vi "AR Drone - Simple Video + Simple nav.vi"() -> ()   [LabVIEW 2014]
doc: "Very simple example showing how to use the base VIs to control the AR Drone and receive and display video data."
uses:
  Others (.ctl)/Control cluster.ctl
  <vilib>/LVH/AR Drone Toolkit/Decode NavData/Typedefs/NavData Demo.ctl
  Global.vi
  <vilib>/LVH/AR Drone Toolkit/AR Drone.lvlib
panel:
  in  "video refresh (ms)":u32
  out "Refesh Rate Video Loop (ms) 2":u32
  in  "Video":bool
  out "Refesh Rate (ms)":u32
  out "Hover":bool
  in  "Tab Control":enum32{"Page 1", "Page 2"}(tab)=enum."Page 2"
  out "Image":T1(plugin-control)
  out "Video Stream 2":picture
  in  "Manual":bool=TRUE
  in  "Takeoff/Land":bool
  in  "Setup Parameters":T2={"Drone IP address"="192.168.1.1", "Home IP address"="192.168.1.2", "Flight Mode"=enum."INDOOR MODE", "Mounted Hull"=enum."INDOOR HULL", "Video Camera"=0, "Max Altitude (m)"=3.0, "Max Pitch and Roll Angle (deg)"=10.0, "Max Vertical Speed (m/s)"=0.7, "Max Yaw Speed (deg/s)"=100.0} {"Video Camera" items=["Bottom Camera"=1, "Front Camera"=0, "Front in Bottom"=3, "Bottom in Front"=2]}
  in  "stop":bool
  in  "milliseconds to wait":u32=5
  out "ctr+nav":errorcluster
  out "ctr+nav":i32=8650
  out "Battery Remaining 2":dbl(slide)=38.0 scale=0.0..100.0
  out "NavData Out 2":T3={"control state"=enum."TRANS_LANDING", "battery percentage"=38, "pitch (deg)"=0.254, "roll (deg)"=0.004, "yaw (deg)"=-28.462, "altitude (cm)"=0, "vx (cm/s)?"=0.0, "vy (cm/s)?"=0.0, "vz (cm/s)?"=0.0, "detection cam type"=3}
  out "Control Cluster":T4={"Roll"=-0.03756714, "Pitch"=-0.007873535, "Vertical Speed"=-0.0, "Yaw Speed"=0.01574707} {"Yaw Speed" scale=-1.0..1.0; "Vertical Speed" scale=-1.0..1.0; "Pitch" scale=-1.0..1.0; "Roll" scale=-1.0..1.0}
  in  "Emergency Landing":bool
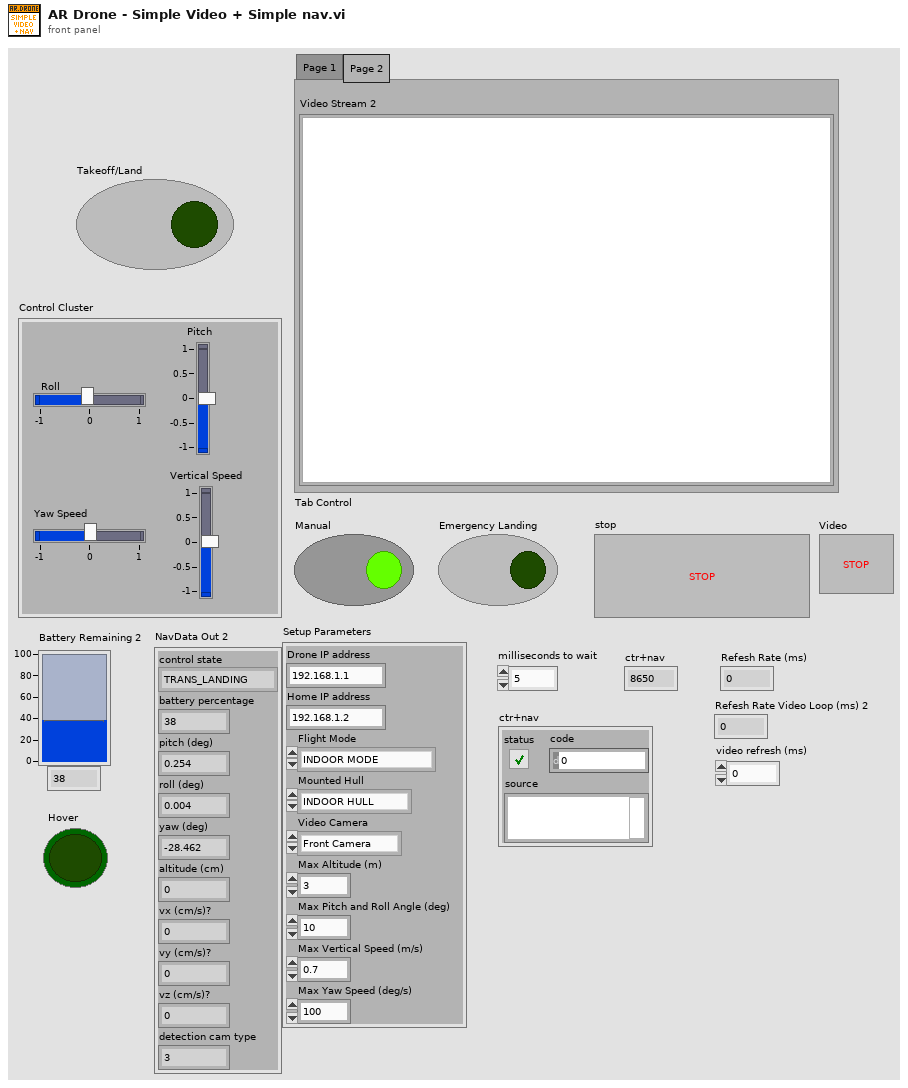
[diagram p1: front panel]
types:
  T1 = typedef "IMAQ Image.ctl" = refnum<image>
  T2 = cluster{"Drone IP address":string, "Home IP address":string, "Flight Mode":enum8{"OUTDOOR MODE", "INDOOR MODE"}, "Mounted Hull":enum8{"OUTDOOR HULL", "INDOOR HULL"}, "Video Camera":u8, "Max Altitude (m)":sgl, "Max Pitch and Roll Angle (deg)":sgl, "Max Vertical Speed (m/s)":sgl, "Max Yaw Speed (deg/s)":sgl}
  T3 = typedef "AR Drone.lvlib/NavData Demo.ctl" = cluster{"control state":enum32{"DEFAULT", "INIT", "LANDING", "FLYING", "HOVERING", "TEST", "TRANS_TAKEOFF", "TRANS_GOTOFIX", "TRANS_LANDING"}, "battery percentage":u32, "pitch (deg)":sgl, "roll (deg)":sgl, "yaw (deg)":sgl, "altitude (cm)":u32, "vx (cm/s)?":sgl, "vy (cm/s)?":sgl, "vz (cm/s)?":sgl, "detection cam type":u32}
  T4 = typedef "Control cluster.ctl" = cluster{"Roll":sgl, "Pitch":sgl, "Vertical Speed":sgl, "Yaw Speed":sgl}
  T5 = typedef "AR Drone.lvlib/AR Drone Resource.ctl" = cluster{"UDP Control Connection":refnum<k16>, "UDP NavData Connection":refnum<k16>, "UDP Video Connection (Drone 1.0)":refnum<k16>, "TCP Video Connection (Drone 2.0)":refnum<k5>, "TCP Control Port Connection":refnum<k5>, "Drone IP address":string, "Drone Command Port":u16, "Drone NavData Port":u16, "Drone Vid Stream Port":u16, "Drone TCP Control Port":u16, "Home IP address":string, "Home Command Port":u16, "Home NavData Port":u16, "Home Vid Stream Port":u16, "Drone Version":i32, "Drone Index":i32, "Command Sequence":i32}
  T6 = cluster{"button 1":bool, "button 2":bool, "button 3":bool, "button 4":bool}
  T7 = cluster{"Roll":dbl, "Pitch":dbl, "Vertical Speed":dbl, "Yaw Speed":dbl}
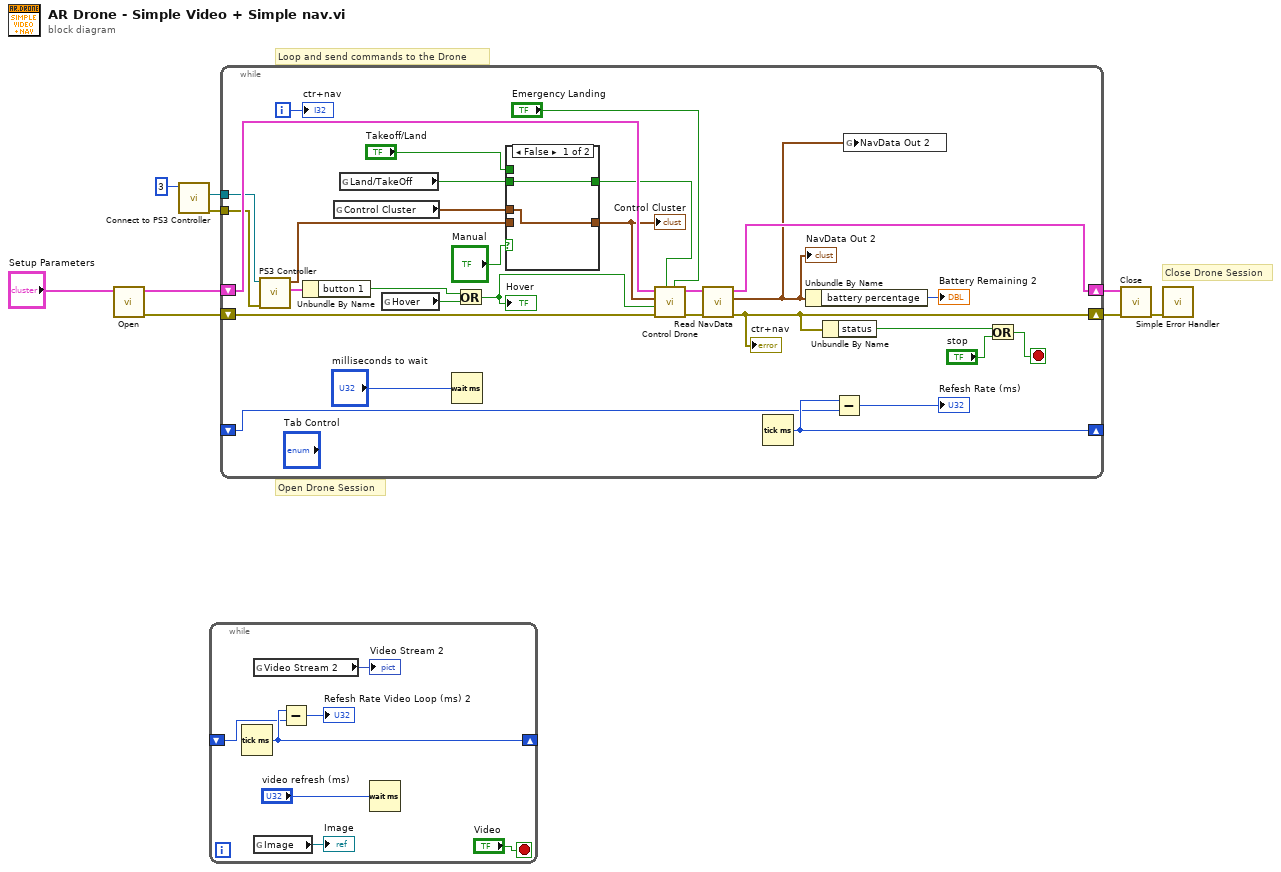
[diagram p0: block diagram]
diagram:
  # "Close Drone Session"
  # "Loop and send commands to the Drone"
  # "Open Drone Session"
  n1 = call <vilib>:"Open.vi"("Setup Parameters"="Setup Parameters") -> ("error out"=w7:errorcluster, "AR Drone Resource"=w3:T5)  [unwired: 9 in]
  n2 = call "Connect to PS3 Controller.vi"("device ID"=3) -> ("error out"=w4:errorcluster, "device ID 2"=w6:refnum<k1>)  [unwired: 7 in, 1 out]
  n3 = while {
    shift-right: [w12] -> _
    shift-left: _ -> [w11]
    stop <- "Video" stop-if-true
    n4 = Tick Count (ms)() -> (millisecond timer value=w12:u32)
    n5 = global read "Global.vi" "Video Stream 2"() -> (→"Video Stream 2":picture)
    n6 = global read "Global.vi" "Image"() -> (→"Image":T1)
    n7 = Subtract(x=w12, y=w11) -> (x-y=→"Refesh Rate Video Loop (ms) 2":u32)
    n8 = Wait (ms)(milliseconds to wait="video refresh (ms)") -> ()  [unwired: 1 out]
  }
  n9 = while {
    shift-right: [w45] -> w9
    shift-left: w3 -> [w42]
    shift-right: [w37] -> w2
    shift-left: w7 -> [w43]
    tunnel: w6 -> [w40]
    tunnel: w4 -> [w39]
    shift-right: [w24] -> _
    shift-left: _ -> [w23]
    i -> [w41]
    stop <- w38 stop-if-true
    n10 = call "PS3 Controller.vi"("error in (no error)"=w39, "device ID"=w40) -> ("Buttons control"=w34:T6, "Control cluster"=w30:T7)  [unwired: 6 in, 2 out]
    n11 = Unbundle By Name(w34) -> ("button 1"=w26:bool)
    n12 = global read "Global.vi" "Control Cluster"() -> (w29:T4)
    n13 = global read "Global.vi" "Land/TakeOff"() -> (w18:bool)
    n14 = global read "Global.vi" "Hover"() -> (w21:bool)
    n15 = Wait (ms)(milliseconds to wait="milliseconds to wait") -> ()  [unwired: 1 out]
    n16 = Or(x=w26, y=w21) -> (x .or. y?=w25:bool)
    "Hover" <- w25
    n17 = case shown="False" "Manual" {
      tunnel: w30 -> [_ w49]
      tunnel: w29 -> [w47 _]
      tunnel: [w47 w49] -> w27
      tunnel: "Takeoff/Land" -> [_ w50]
      tunnel: [w48 w50] -> w19
      tunnel: w18 -> [w48 _]
      frame False {
      }
      frame True {
      }
    }
    "Control Cluster" <- w27
    n18 = call <vilib>:"Control Drone.vi"("Emergency Landing"="Emergency Landing", "Takeoff/Land"=w19, "error in (no error)"=w43, "Hover"=w25, "Control Cluster"=w27, "AR Drone Resource"=w42) -> ("error out"=w32:errorcluster, "AR Drone Resource Out"=w33:T5)  [unwired: 4 in]
    n19 = call <vilib>:"Read NavData.vi"("error in (no error)"=w32, "AR Drone Resource"=w33) -> ("error out"=w37:errorcluster, "NavData Out"=w17:T3, "AR Drone Resource Out"=w45:T5)  [unwired: 7 in]
    "ctr+nav" <- w37
    "NavData Out 2" <- w17
    n20 = Tick Count (ms)() -> (millisecond timer value=w24:u32)
    n21 = Unbundle By Name(w17) -> ("battery percentage"=→"Battery Remaining 2":u32)
    n22 = Unbundle By Name(w37) -> ("status"=w35:bool)
    n23 = Subtract(x=w24, y=w23) -> (x-y=→"Refesh Rate (ms)":u32)
    n24 = global write "Global.vi" "NavData Out 2"(w17) -> ()
    n25 = Or(x=w35, y="stop") -> (x .or. y?=w38:bool)
    "ctr+nav" <- w41
  }
  n26 = call <vilib>:"Close.vi"("error in (no error)"=w2, "AR Drone Resource"=w9) -> ("error out"=w8:errorcluster)  [unwired: 9 in]
  n27 = call <vilib>:"Simple Error Handler.vi"("error in (no error)"=w8) -> ()  [unwired: 4 in, 5 out]
